vi "Command Finished.vi"(8 "error in (no error)":errorcluster, 10 "Command Name (Instance)":string, 11 "Running Command in":refnum<class "Running Command.lvclass">) -> (0 "error out":errorcluster, 3 "Running Command out":refnum<class "Running Command.lvclass">)   [LabVIEW 2014, in "Robot Actor Framework.lvlib" / "Command Processor Actor.lvlib" / "Running Command.lvclass"]
uses:
  Running Command.lvclass
  <vilib>/ActorFramework/Message Enqueuer/Message Priority.ctl
  <vilib>/ActorFramework/Actor/Actor.lvclass/Actor.ctl
  <vilib>/ActorFramework/Message Enqueuer/Message Enqueuer.lvclass/Message Enqueuer.ctl
  <vilib>/ActorFramework/Message Enqueuer/Init from Existing Queue.vi
  <vilib>/ActorFramework/Message Enqueuer/Enqueue.vi
  <vilib>/ActorFramework/Message Priority Queue/Priority Enqueue.vi
  Command Processor Actor Class/Command Processor Actor.lvclass
  <vilib>/ActorFramework/Message Enqueuer/Message Enqueuer.lvclass
  Command Processor Actor Messages/Go To Finishing Command Msg/Go To Finishing Command Msg.lvclass
  <vilib>/ActorFramework/Actor/Actor.lvclass
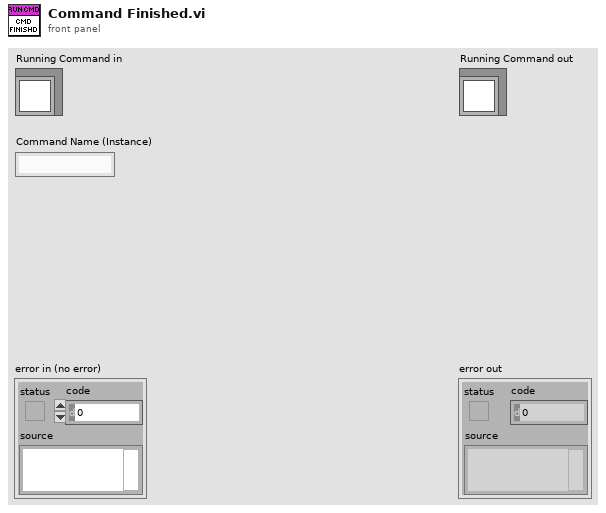
[diagram p1: front panel]
types:
  T1 = typedef "Actor Framework.lvlib/Message Enqueuer.lvclass/Message Priority.ctl" = enum16{"Low", "Normal", "High"}
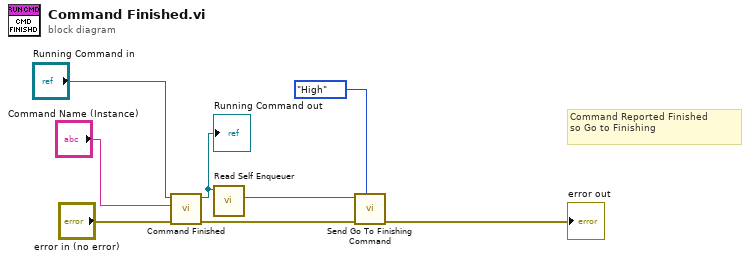
[diagram p0: block diagram]
diagram:
  # "Command Reported Finished\nso Go to Finishing"
  n1 = call-parent "Command Finished.vi"("error in (no error)"="error in (no error)", "Command Name (Instance)"="Command Name (Instance)", "Command Processor in"="Running Command in") -> ("error out"=w4:errorcluster, "Command Processor out"=w8:refnum<class "Running Command.lvclass">)  [unwired: 7 in]
  "Running Command out" <- w8
  n2 = call <vilib>:"Read Self Enqueuer.vi"("Actor"=w8) -> ("Self Enqueuer"=w5:refnum<class "Message Enqueuer.lvclass">)  [unwired: 10 in]
  n3 = call "Send Go To Finishing Command.vi"("Message Priority (Normal)"=Message_Priority."High", "error in (no error)"=w4, "Message Enqueuer"=w5) -> ("error out"=→"error out":errorcluster)  [unwired: 7 in, 1 out]
